vi "GetTurnDirection.vi"(9 "Target Angle":dbl, 11 "Robot Angle":dbl) -> (3 "Numeric":dbl)   [LabVIEW 2018]
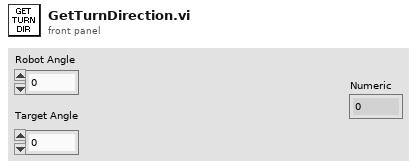
[diagram p1: front panel]
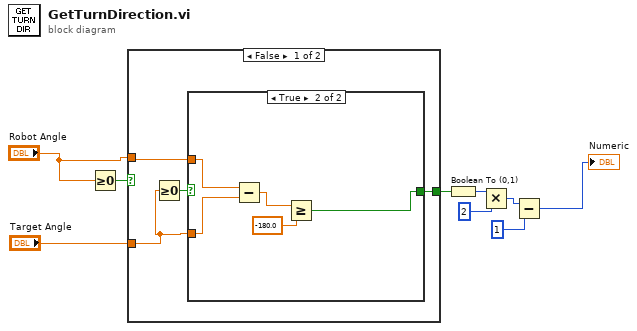
[diagram p0: block diagram]
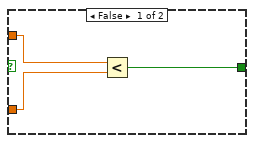
[diagram p2: hidden frame]
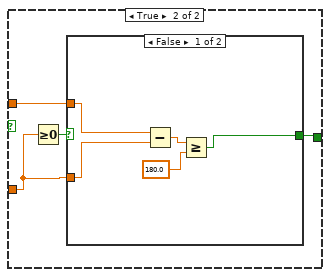
[diagram p3: hidden frame]
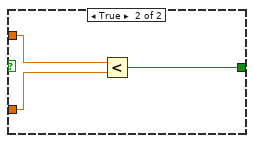
[diagram p4: hidden frame]
diagram:
  n1 = Greater Or Equal To 0?(x="Robot Angle") -> (x >= 0?=w9:bool)
  n2 = case shown="False" w9 {
    tunnel: "Robot Angle" -> [w11 w24]
    tunnel: "Target Angle" -> [w10 w23]
    tunnel: [w12 w22] -> w6
    frame False {
      n3 = Greater Or Equal To 0?(x=w10) -> (x >= 0?=w13:bool)
      n4 = case shown="True" w13 {
        tunnel: w11 -> [w16 w21]
        tunnel: w10 -> [w15 w20]
        tunnel: [w14 w17] -> w12
        frame False {
          n5 = Less?(x=w16, y=w15) -> (x < y?=w14:bool)
        }
        frame True {
          n6 = Subtract(x=w21, y=w20) -> (x-y=w19:dbl)
          n7 = Greater Or Equal?(x=w19, y=-180.0) -> (x >= y?=w17:bool)
        }
      }
    }
    frame True {
      n8 = Greater Or Equal To 0?(x=w23) -> (x >= 0?=w25:bool)
      n9 = case shown="False" w25 {
        tunnel: w24 -> [w30 w33]
        tunnel: w23 -> [w29 w32]
        tunnel: [w26 w31] -> w22
        frame False {
          n10 = Subtract(x=w30, y=w29) -> (x-y=w28:dbl)
          n11 = Greater Or Equal?(x=w28, y=180.0) -> (x >= y?=w26:bool)
        }
        frame True {
          n12 = Less?(x=w33, y=w32) -> (x < y?=w31:bool)
        }
      }
    }
  }
  n13 = Boolean To (0,1)(Boolean=w6) -> (0, 1=w5:i16)
  n14 = Multiply(x=w5, y=i16 2) -> (x*y=w3:i16)
  n15 = Subtract(x=w3, y=i16 1) -> (x-y=→"Numeric":i16)
